vi "Hold_open.vi"   [LabVIEW 2010]
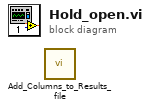
[diagram p0: block diagram]
diagram:
  n1 = call "Add_Columns_to_Results_file.vi"() -> ()  [unwired: 5 in, 5 out]
